vi "TestCloneAPI.vi"() -> ()   [LabVIEW 2014, in "NetworkImpairmentModule.lvlib"]
uses:
  NetworkImpairmentModule.lvlib
  PublicAPI/Arguments/Requests/dblTimeArray.ctl
  PublicAPI/Arguments/Requests/dblNetImpParams.ctl
  PublicAPI/Arguments/Requests/dblLossThreshold.ctl
  PublicAPI/Arguments/Broadcasts/dblNetworkTime.ctl
  PublicAPI/Arguments/Broadcasts/dblPktLoss.ctl
  <userlib>/NIST/ModuleAdminLib/ModuleAdmin/ModuleAdmin.lvclass
  PublicAPI/Arguments/Broadcasts/clDidInit.ctl
  <userlib>/NIST/ModuleAdminLib/ModuleAdmin/ModuleAdmin.lvclass/ModuleAdmin.ctl
  PublicAPI/Arguments/Requests/clStopArgument.ctl
  PublicAPI/Arguments/Broadcasts/clStatUpdate.ctl
  PublicAPI/Arguments/Broadcasts/clErrorRpt.ctl
  <userlib>/NIST/ModuleAdminLib/ModuleAdmin/Accessors/Read CloneRegRef.vi
  <vilib>/Analysis/1siggen.llb/Ramp Pattern by Delta.vi
  <userlib>/NIST/ModuleAdminLib/CloneRegistration/CloneRegistration.lvclass
  <vilib>/Analysis/NI_AALBase.lvlib
panel:
  in  "Show Panel":bool=TRUE
  out "PluginPathReport":path
  in  "btnReadPathToNetImpairPlugin":bool
  in  "btnLoadNetImpairPlugin":bool
  in  "PluginPath":path=path "P:/Framework/NetworkImpairment/NetworkImpairmentPlugins/NetworkPlugin/NetworkPlugin.ini"
  in  "Delta":dbl=60.0
  in  "End":dbl=10.0
  in  "Start":dbl
  in  "btnGetPktLoss":bool
  in  "btnGetNetTime":bool
  out "dblPktLoss":T1
  out "dblNetTime":T2
  in  "btnReadLossThreshold":bool
  out "dblLossThresholdReport":T3
  in  "btnWriteLossThreshold":bool
  in  "dblLossThreshold":T3
  in  "btnReadNetImpParams":bool
  out "dblNetImpParamsReport":T4
  in  "btnWriteNetImpParams":bool
  in  "dblNetImpParams":T4=[[0.5], [0.1], [0.03], [0.95], [5.0]]
  in  "dblTimeArray":T5
  in  "btnWriteTime":bool
  in  "btnRemove":bool
  out "Status Log":string
  out "Active Modules (Array)":string[](array[string])
  in  "btnAdd":bool
  in  "btnStop":bool
  in  "Select Module":i32(ring)=-1 caption="Select Module to send Request" items=["All"=-1, "4140002"=4140002, "4140003"=4140003, "4140004"=4140004, "4140005"=4140005]
  # "Hidden"
  # "Visible"
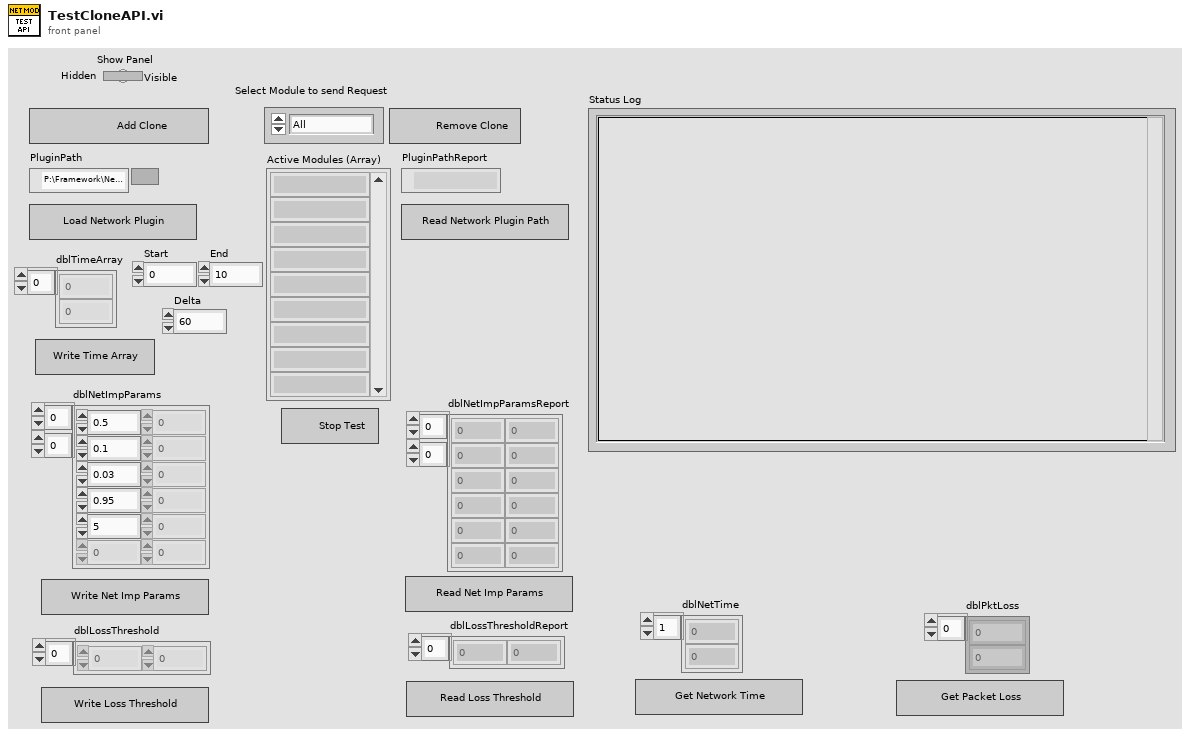
[diagram p1: front panel]
types:
  T1 = typedef "NetworkImpairmentModule.lvlib/dblPktLoss.ctl" = dbl[]
  T2 = typedef "NetworkImpairmentModule.lvlib/dblNetworkTime.ctl" = dbl[]
  T3 = typedef "NetworkImpairmentModule.lvlib/dblLossThreshold.ctl" = dbl[]
  T4 = typedef "NetworkImpairmentModule.lvlib/dblNetImpParams.ctl" = dbl[][]
  T5 = typedef "NetworkImpairmentModule.lvlib/dblTimeArray.ctl" = dbl[]
  T6 = typedef "NetworkImpairmentModule.lvlib/clBroadcastEvents.ctl" = cluster{"DidInit":refnum<user-event>, "StatusUpdate":refnum<user-event>, "ErrorReport":refnum<user-event>, "DidStop":refnum<user-event>, "ReadNetImpParams":refnum<user-event>, "ReadLossThreshold":refnum<user-event>, "GetNetworkTime":refnum<user-event>, "GetPktLoss":refnum<user-event>, "ReadPathToPlugin":refnum<user-event>}
  T7 = typedef "NetworkImpairmentModule.lvlib/clDidInit.ctl" = cluster{"Init?":bool, "ModuleAdmin":refnum<class "ModuleAdmin.lvclass">}
  T8 = typedef "NetworkImpairmentModule.lvlib/clStopArgument.ctl" = cluster{"Exit via Stop Module Req?":bool, "Wait for Module to stop?":bool, "ModuleAdmin":refnum<class "ModuleAdmin.lvclass">}
  T9 = typedef "NetworkImpairmentModule.lvlib/clStatUpdate.ctl" = cluster{"Status":string}
  T10 = typedef "NetworkImpairmentModule.lvlib/clErrorRpt.ctl" = cluster{"error":errorcluster, "AdditionalInfo":string}
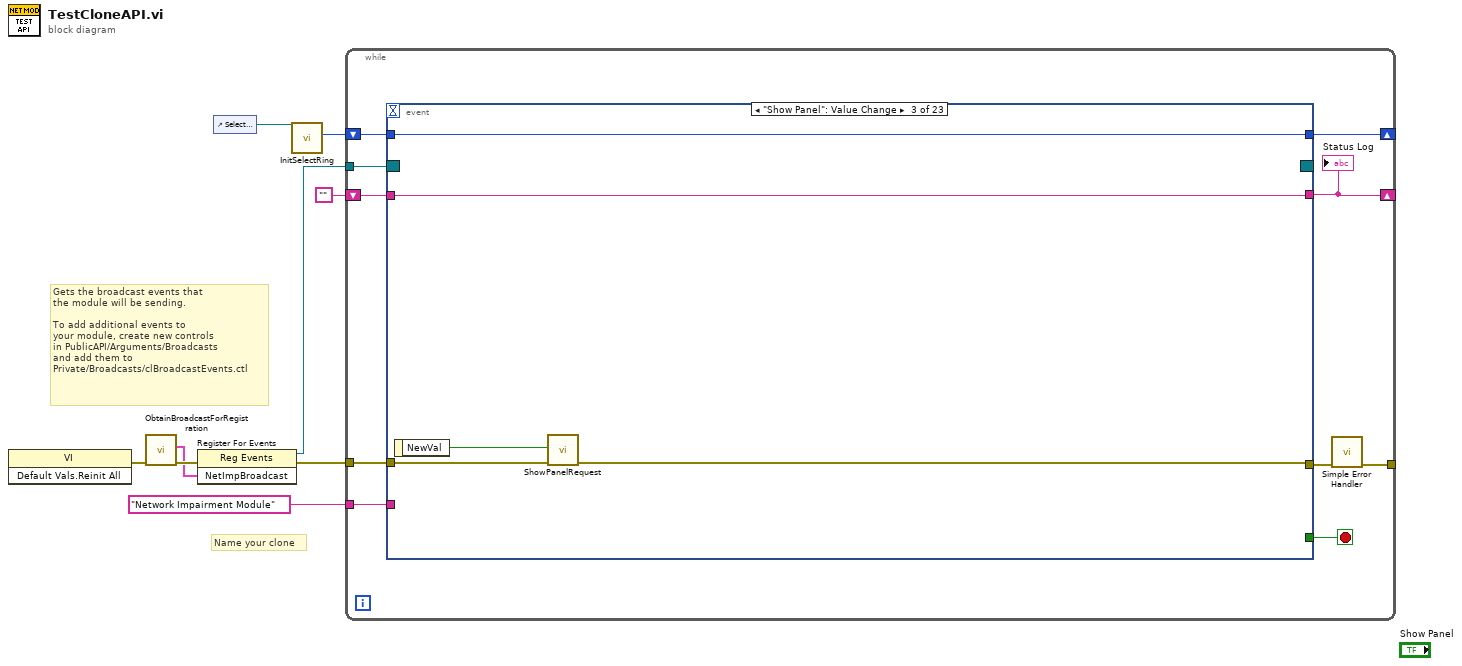
[diagram p0: block diagram]
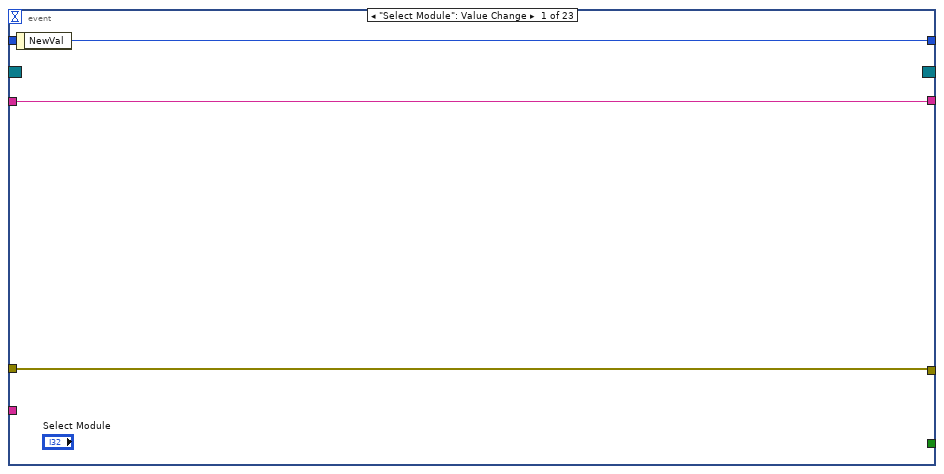
[diagram p2: hidden frame]
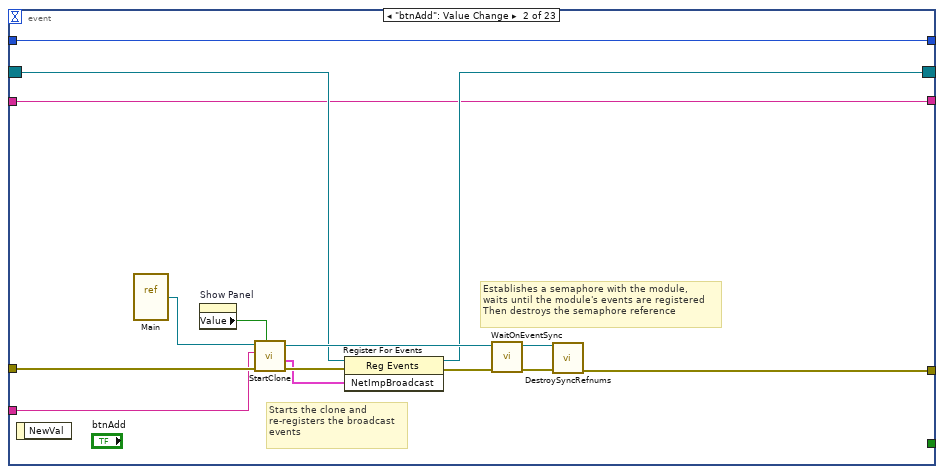
[diagram p3: hidden frame]
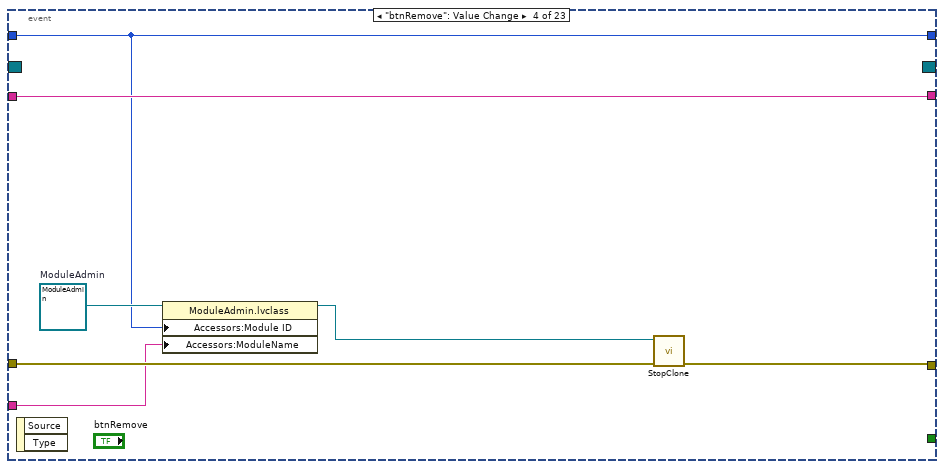
[diagram p4: hidden frame]
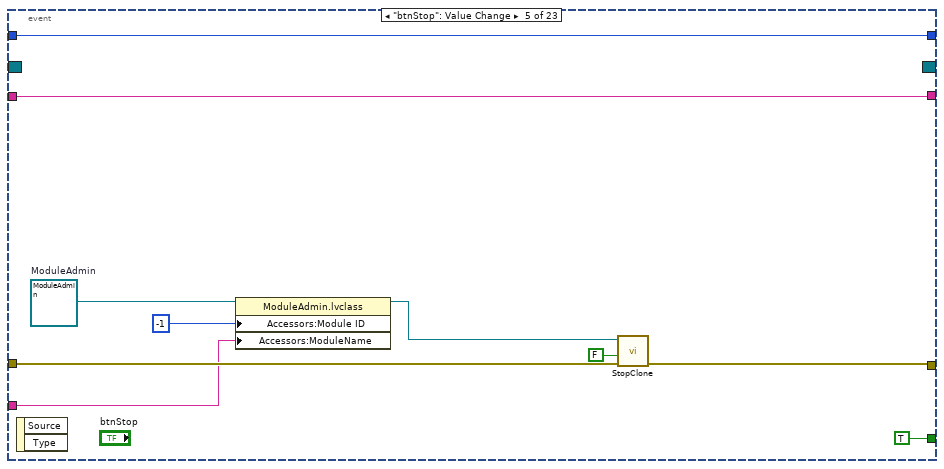
[diagram p5: hidden frame]
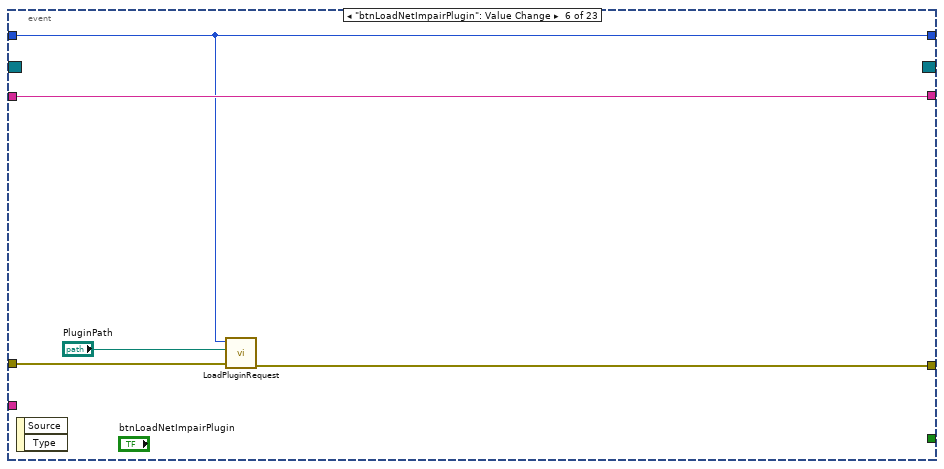
[diagram p6: hidden frame]
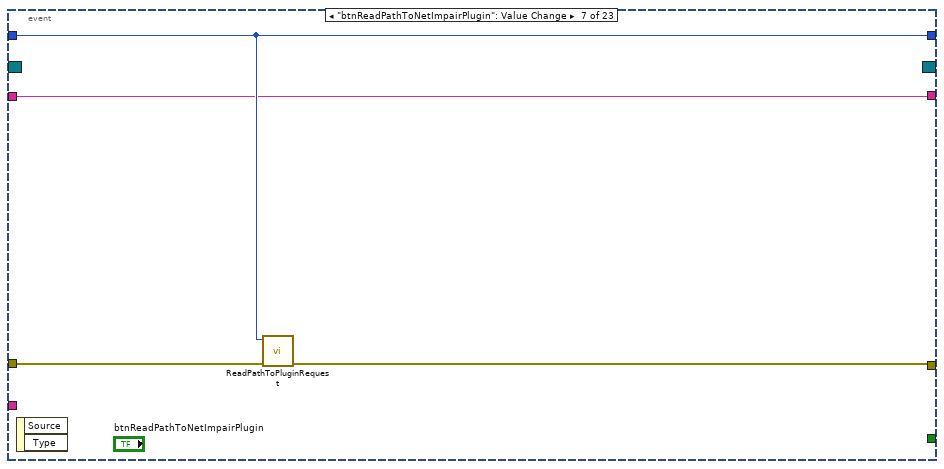
[diagram p7: hidden frame]
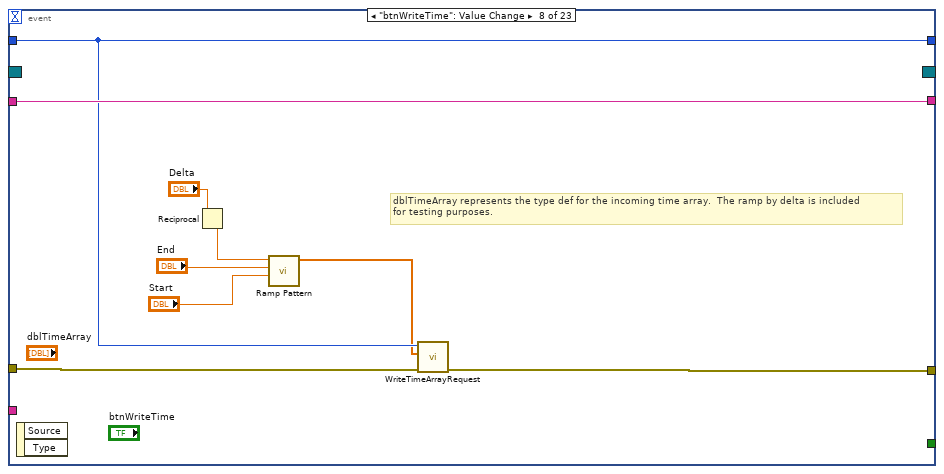
[diagram p8: hidden frame]
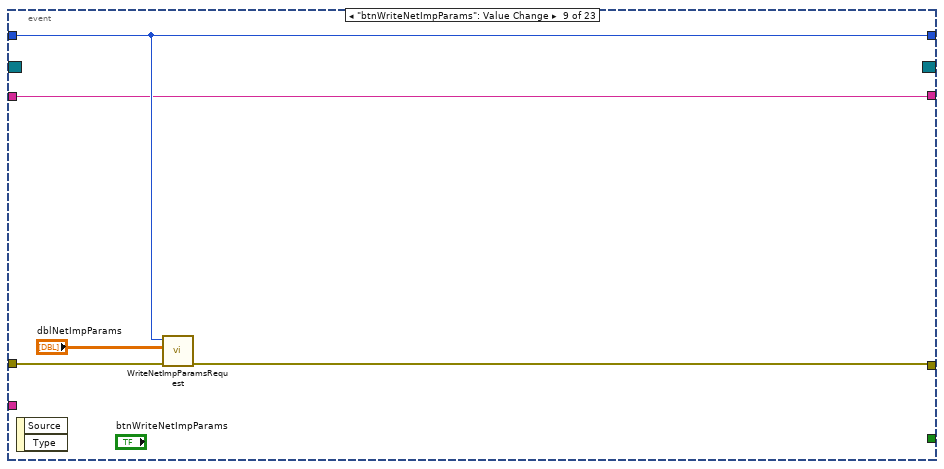
[diagram p9: hidden frame]
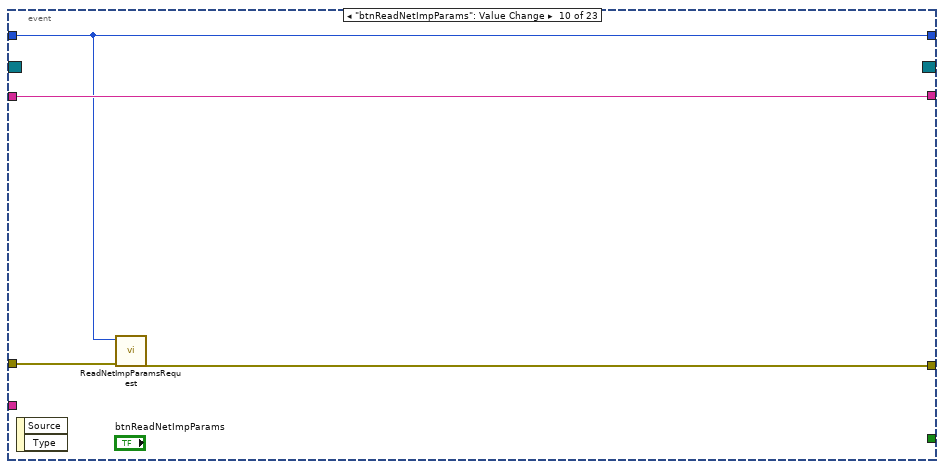
[diagram p10: hidden frame]
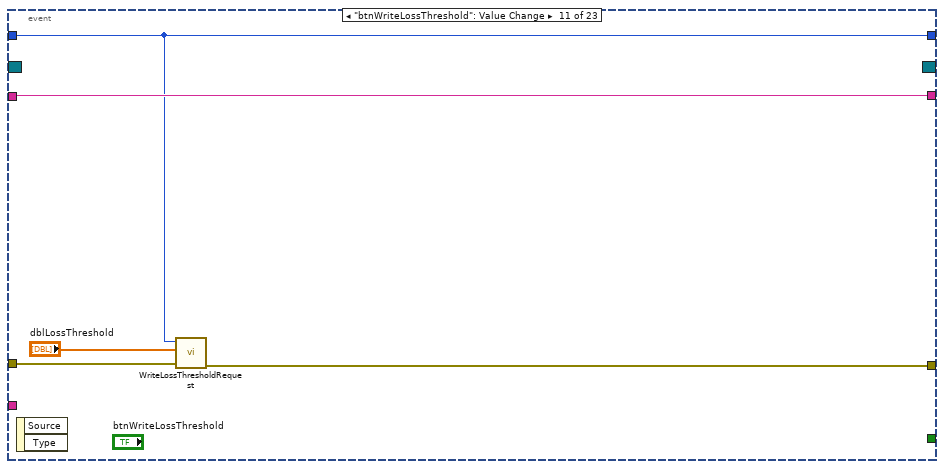
[diagram p11: hidden frame]
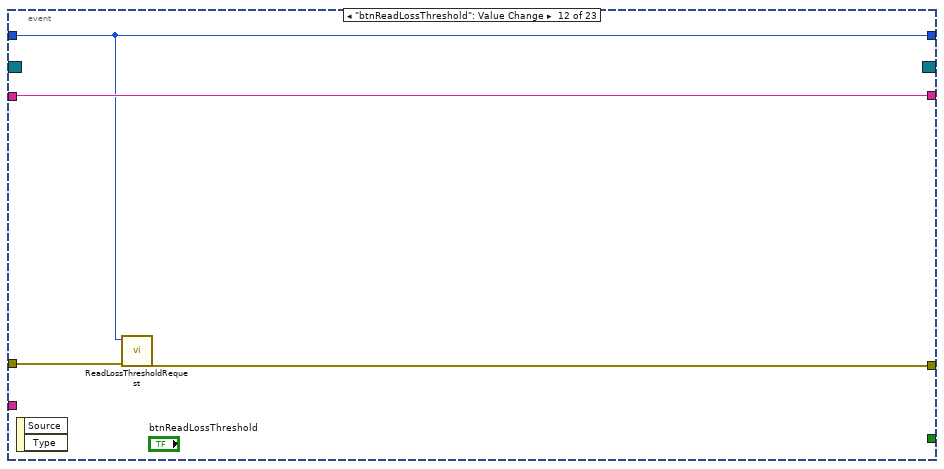
[diagram p12: hidden frame]
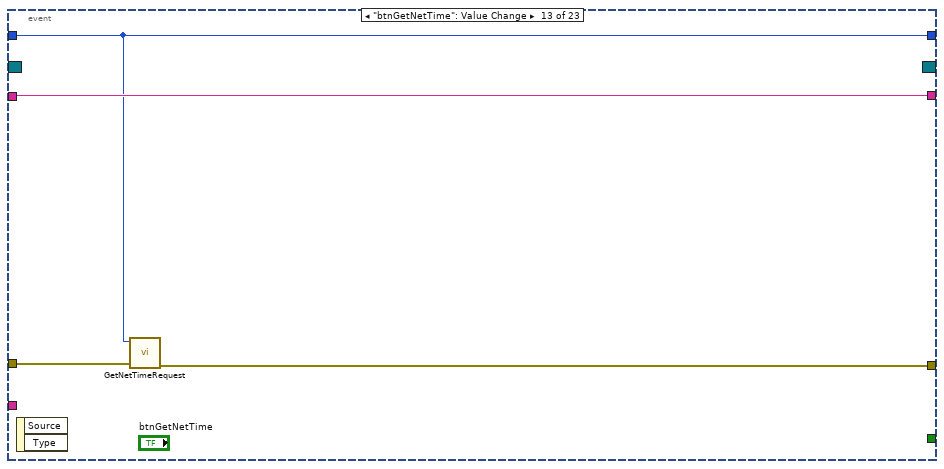
[diagram p13: hidden frame]
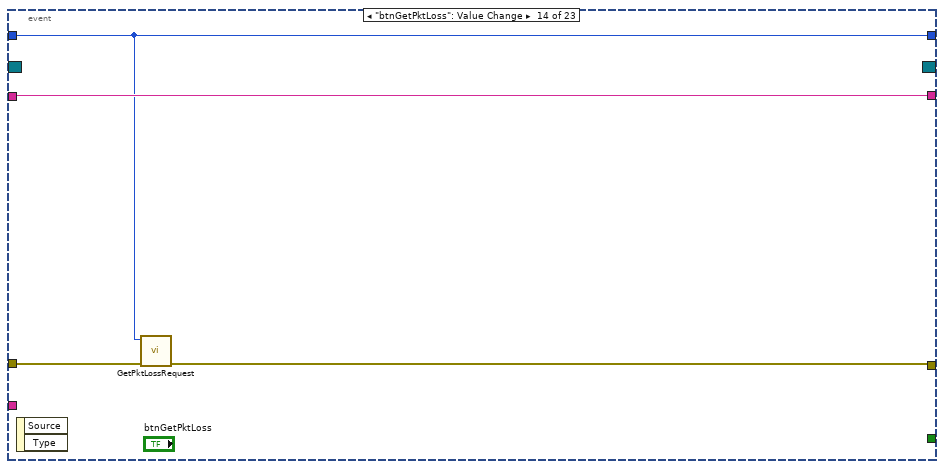
[diagram p14: hidden frame]
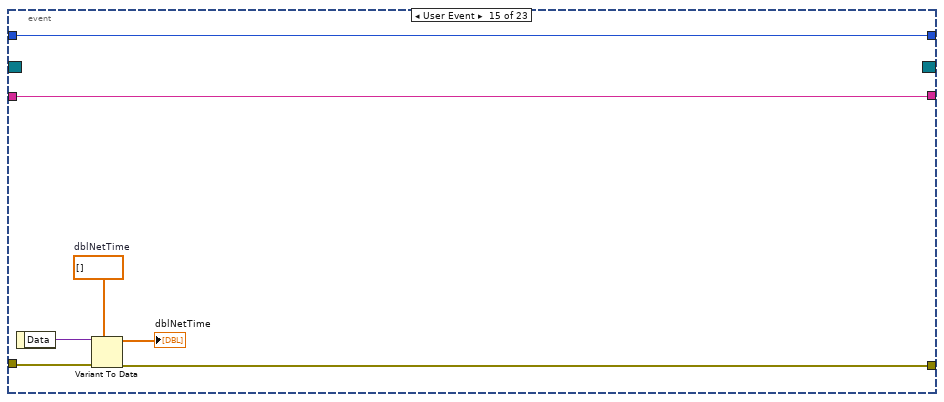
[diagram p15: hidden frame]
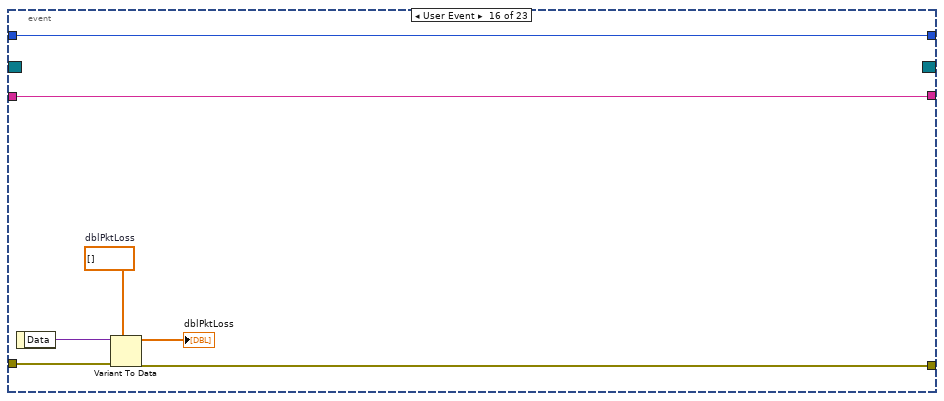
[diagram p16: hidden frame]
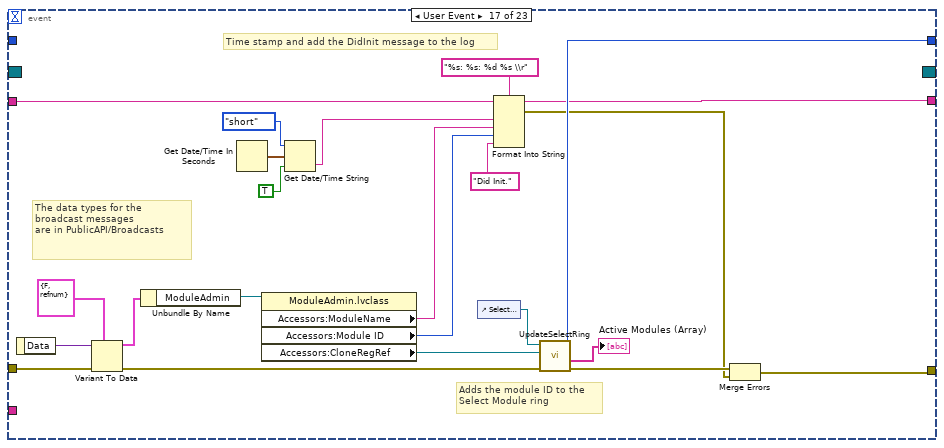
[diagram p17: hidden frame]
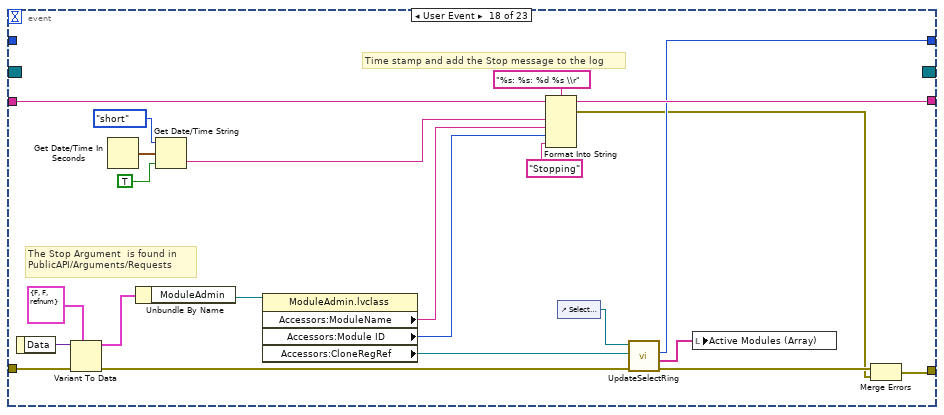
[diagram p18: hidden frame]
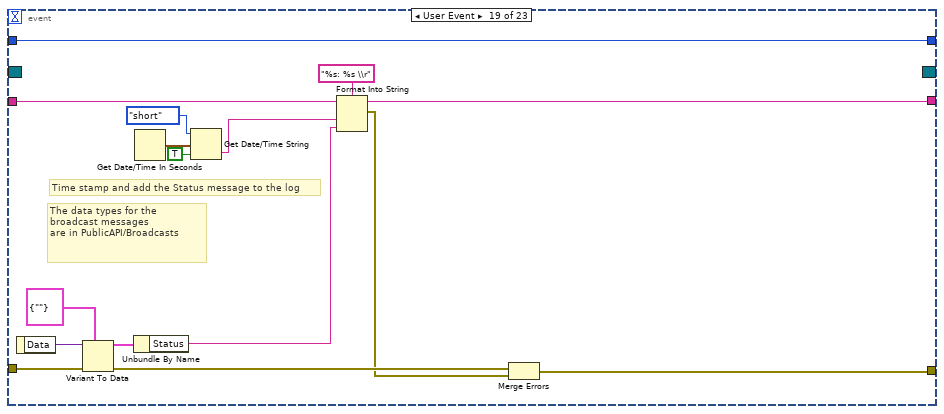
[diagram p19: hidden frame]
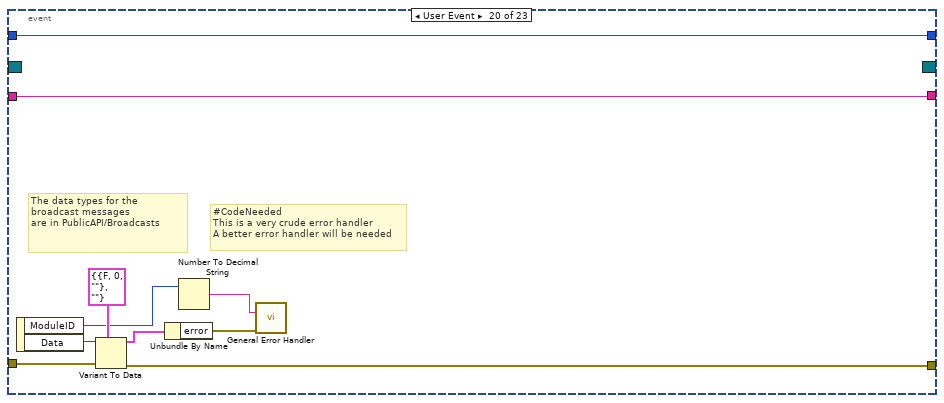
[diagram p20: hidden frame]
diagram:
  # "Name your clone"
  # "Gets the broadcast events that\nthe module will be sending.\n\nTo add additional events to\nyour module, create new controls\nin PublicAPI/Arguments/Broadcasts\nand add them to\nPrivate/Broadcasts/clBroadcastEvents.ctl"
  n1 = invoke class="VI" method="Default Vals.Reinit All"() -> (error out=w7:errorcluster)  [unwired: 3 in, 2 out]
  n2 = call "ObtainBroadcastForRegistration.vi"("error in (no error)"=w7) -> ("error out"=w6:errorcluster, "NetImpBroadcast"=w5:T6)  [unwired: 9 in]
  n3 = register-events(error in=w6, w5) -> (reference out=w3:refnum<event-registration>, error out=w4:errorcluster)  [unwired: 1 in]
  n4 = control-ref of="Select Module"() -> (w9:refnum<vi>)
  n5 = call "InitSelectRing.vi"("Ring Refnum"=w9) -> ("Module Ring Value"=w8:i32)  [unwired: 9 in, 1 out]
  n6 = while {
    shift-right: [w18] -> _
    shift-left: w8 -> [w19]
    tunnel: w4 -> [w16]
    tunnel: w3 -> [w13]
    tunnel: [w14] -> _
    shift-right: [w12] -> _
    shift-left: "" -> [w11]
    tunnel: "Network Impairment Module" ("ModuleName") -> [w10]
    stop <- w17 stop-if-true
    n7 = event shown="[2] \"Show Panel\": Value Change" {
      selector: w13 -> [_ w28 _ _ _ _ _ _ _ _ _ _ _ _ _ _ _ _ _ _ _ _ _]
      dyn-events: [_ w27 _ _ _ _ _ _ _ _ _ _ _ _ _ _ _ _ _ _ _ _ _] -> _
      timeout: _ -> [_ _ _ _ _ _ _ _ _ _ _ _ _ _ _ _ _ _ _ _ _ _ _]
      tunnel: w19 -> [_ w37 w41 w44 w59 w60 w66 w75 w80 w83 w87 w92 w96 w100 w104 w111 _ _ w179 w181 w192 w197 w205]
      tunnel: [w22 w37 w41 w44 w59 w60 w66 w75 w80 w83 w87 w92 w96 w100 w104 w111 w135 w150 w179 w181 w192 w197 w205] -> w18
      tunnel: [_ _ _ _ TRUE _ _ _ _ _ _ _ _ _ _ _ _ _ _ _ _ _ _] -> w17
      tunnel: w16 -> [w20 w36 w40 w48 w57 w63 w68 w76 w82 w86 w91 w95 w99 w103 w110 w117 w140 w159 w176 w188 w195 w202 w210]
      tunnel: [w20 w29 w38 w47 w55 w62 w67 w74 w78 w85 w90 w94 w98 w102 w107 w114 w124 w147 w167 w187 w194 w201 w208] -> w15
      tunnel: [w21 w25 w42 w49 w54 w64 w65 w77 w79 w84 w89 w93 w97 w101 w105 w112 w128 w156 w170 w180 w191 w198 w204] -> w12
      tunnel: w11 -> [w21 w25 w42 w49 w54 w64 w65 w77 w79 w84 w89 w93 w97 w101 w105 w112 w127 w157 w178 w180 w191 w198 w204]
      tunnel: w10 -> [_ w24 _ w45 w51 _ _ _ _ _ _ _ _ _ _ _ _ _ _ _ _ _ _]
      event "Select Module": Value Change {
        n8 = event-data() -> ("NewVal"=w22:i32)  [unwired: 1 in]
      }
      event "btnAdd": Value Change {
        # "Establishes a semaphore with the module,\nwaits until the module's events are registered\nThen destroys the semaphore reference"
        # "Starts the clone and\nre-registers the broadcast \nevents"
        n9 = event-data() -> ()  [unwired: 1 in, 1 out]
        n10 = vi-ref "Main.vi"() -> (w26:refnum<vi>)
        n11 = property on="Show Panel" class="Bool (strict)"() -> ("Value"=w23:bool)  [unwired: 2 in, 2 out]
        n12 = call "StartClone.vi"("ShowPanel? (f)"=w23, "error in (no error)"=w36, "ModuleName"=w24, "VI Refnum"=w26) -> ("error out"=w35:errorcluster, "clBroadcastEvents"=w30:T6, "ModuleAdmin"=w32:refnum<class "ModuleAdmin.lvclass">)  [unwired: 5 in]
        n13 = register-events(reference=w28, error in=w35, w30) -> (reference out=w27:refnum<event-registration>, error out=w34:errorcluster)
        n14 = call <userlib>:"WaitOnEventSync.vi"("error in (no error)"=w34, "ModuleAdmin"=w32) -> ("error out"=w33:errorcluster, "ModuleAdmin"=w31:refnum<class "ModuleAdmin.lvclass">)  [unwired: 8 in]
        n15 = call <userlib>:"DestroySyncRefnums.vi"("error in (no error)"=w33, "ModuleAdmin"=w31) -> ("error out"=w29:errorcluster)  [unwired: 9 in]
      }
      event "Show Panel": Value Change {
        n16 = event-data() -> ("NewVal"=w39:bool)  [unwired: 1 in]
        n17 = call "ShowPanelRequest.vi"("error in (no error)"=w40, "ShowPanel?"=w39) -> ("error out"=w38:errorcluster)  [unwired: 9 in]
      }
      event "btnRemove": Value Change {
        w46 = refnum<class "ModuleAdmin.lvclass"> refnum  # ModuleAdmin
        n18 = event-data() -> ()  [unwired: 1 in, 2 out]
        n19 = property class="ModuleAdmin.lvclass"(reference=w46, "Accessors:Module ID"=w44, "Accessors:ModuleName"=w45) -> (reference out=w43:refnum<class "ModuleAdmin.lvclass">)  [unwired: 1 in, 1 out]
        n20 = call "StopClone.vi"("error in (no error)"=w48, "ModuleAdmin"=w43) -> ("error out"=w47:errorcluster)  [unwired: 9 in]
      }
      event "btnStop": Value Change {
        w53 = refnum<class "ModuleAdmin.lvclass"> refnum  # ModuleAdmin
        n21 = event-data() -> ()  [unwired: 1 in, 2 out]
        n22 = property class="ModuleAdmin.lvclass"(reference=w53, "Accessors:Module ID"=-1 ("Module ID"), "Accessors:ModuleName"=w51) -> (reference out=w50:refnum<class "ModuleAdmin.lvclass">)  [unwired: 1 in, 1 out]
        n23 = call "StopClone.vi"("error in (no error)"=w57, "Wait for Module to stop?"=FALSE, "ModuleAdmin"=w50) -> ("error out"=w55:errorcluster)  [unwired: 8 in]
      }
      event "btnLoadNetImpairPlugin": Value Change {
        n24 = event-data() -> ()  [unwired: 1 in, 2 out]
        n25 = call "LoadPluginRequest.vi"("error in (no error)"=w63, "PathToPlugin"="PluginPath", "ModuleID"=w60) -> ("error out"=w62:errorcluster)  [unwired: 8 in]
      }
      event "btnReadPathToNetImpairPlugin": Value Change {
        n26 = event-data() -> ()  [unwired: 1 in, 2 out]
        n27 = call "ReadPathToPluginRequest.vi"("error in (no error)"=w68, "ModuleID"=w66) -> ("error out"=w67:errorcluster)  [unwired: 9 in]
      }
      event "btnWriteTime": Value Change {
        # "dblTimeArray represents the type def for the incoming time array.  The ramp by delta is included\nfor testing purposes."
        n28 = event-data() -> ()  [unwired: 1 in, 2 out]
        n29 = Reciprocal(x="Delta") -> (1/x=w69:dbl)
        n30 = call-poly <vilib>:"Ramp Pattern.vi"("start"="Start", "end"="End", "delta"=w69) -> ("Ramp Pattern"=w70:dbl[])  [unwired: 6 in, 2 out]
        n31 = call "WriteTimeArrayRequest.vi"("error in (no error)"=w76, "TimeArray"=w70, "Module ID"=w75) -> ("error out"=w74:errorcluster)  [unwired: 8 in]
      }
      event "btnWriteNetImpParams": Value Change {
        n32 = event-data() -> ()  [unwired: 1 in, 2 out]
        n33 = call "WriteNetImpParamsRequest.vi"("error in (no error)"=w82, "dblNetImpParams"="dblNetImpParams", "ModuleID"=w80) -> ("error out"=w78:errorcluster)  [unwired: 8 in]
      }
      event "btnReadNetImpParams": Value Change {
        n34 = event-data() -> ()  [unwired: 1 in, 2 out]
        n35 = call "ReadNetImpParamsRequest.vi"("error in (no error)"=w86, "ModuleID"=w83) -> ("error out"=w85:errorcluster)  [unwired: 9 in]
      }
      event "btnWriteLossThreshold": Value Change {
        n36 = event-data() -> ()  [unwired: 1 in, 2 out]
        n37 = call "WriteLossThresholdRequest.vi"("error in (no error)"=w91, "dblLossThreshold"="dblLossThreshold", "ModuleID"=w87) -> ("error out"=w90:errorcluster)  [unwired: 8 in]
      }
      event "btnReadLossThreshold": Value Change {
        n38 = event-data() -> ()  [unwired: 1 in, 2 out]
        n39 = call "ReadLossThresholdRequest.vi"("error in (no error)"=w95, "ModuleID"=w92) -> ("error out"=w94:errorcluster)  [unwired: 9 in]
      }
      event "btnGetNetTime": Value Change {
        n40 = event-data() -> ()  [unwired: 1 in, 2 out]
        n41 = call "GetNetTimeRequest.vi"("error in (no error)"=w99, "ModuleID"=w96) -> ("error out"=w98:errorcluster)  [unwired: 9 in]
      }
      event "btnGetPktLoss": Value Change {
        n42 = event-data() -> ()  [unwired: 1 in, 2 out]
        n43 = call "GetPktLossRequest.vi"("error in (no error)"=w103, "ModuleID"=w100) -> ("error out"=w102:errorcluster)  [unwired: 9 in]
      }
      event User Event {
        w106 = T2 []  # dblNetTime
        n44 = event-data() -> ("Data"=w109:variant)  [unwired: 1 in]
        n45 = Variant To Data(error in=w110, type=w106, Variant=w109) -> (data=→"dblNetTime":T2, error out=w107:errorcluster)
      }
      event User Event {
        w113 = T1 []  # dblPktLoss
        n46 = event-data() -> ("Data"=w116:variant)  [unwired: 1 in]
        n47 = Variant To Data(error in=w117, type=w113, Variant=w116) -> (data=→"dblPktLoss":T1, error out=w114:errorcluster)
      }
      event User Event {
        # "Adds the module ID to the \nSelect Module ring"
        # "Time stamp and add the DidInit message to the log"
        # "The data types for the broadcast messages\nare in PublicAPI/Broadcasts"
        n48 = event-data() -> ("Data"=w139:variant)  [unwired: 1 in]
        n49 = Variant To Data(error in=w140, type=T7 {"Init?"=FALSE, "ModuleAdmin"=refnum} ("clDidInit"), Variant=w139) -> (data=w132:T7, error out=w137:errorcluster)
        n50 = Unbundle By Name(w132) -> ("ModuleAdmin"=w121:refnum<class "ModuleAdmin.lvclass">)
        n51 = Get Date/Time In Seconds() -> (seconds since 1Jan1904=w130:timestamp)
        n52 = property class="ModuleAdmin.lvclass"(reference=w121) -> ("Accessors:ModuleName"=w120:string, "Accessors:Module ID"=w119:i32, "Accessors:CloneRegRef"=w118:refnum<data-value>)  [unwired: 1 in, 2 out]
        n53 = Get Date/Time String(date format (0)=enum16{"short", "long", "abbreviated"}."short", seconds (now)=w130, want seconds? (F)=TRUE) -> (time string=w133:string)  [unwired: 1 out]
        n54 = control-ref of="Select Module"() -> (w136:refnum<vi>)
        n55 = Format Into String(format string="%s: %s: %d %s \\r", initial string=w127, w133, w120, w119, "Did Init.") -> (resulting string=w128:string, error out=w125:errorcluster)  [unwired: 1 in]
        n56 = call "UpdateSelectRing.vi"("error in (no error)"=w137, "CloneRegRef"=w118, "Ring Refnum"=w136) -> ("error out"=w126:errorcluster, "ActiveModules"=→"Active Modules (Array)":string[], "Module Ring Value"=w135:i32)  [unwired: 6 in]
        n57 = Merge Errors(w126, w125) -> (w124:errorcluster)
      }
      event User Event {
        # "Time stamp and add the Stop message to the log"
        # "The Stop Argument  is found in\nPublicAPI/Arguments/Requests"
        n58 = event-data() -> ("Data"=w158:variant)  [unwired: 1 in]
        n59 = Variant To Data(error in=w159, type=T8 {"Exit via Stop Module Req?"=FALSE, "Wait for Module to stop?"=FALSE, "ModuleAdmin"=refnum} ("Stop Argument"), Variant=w158) -> (data=w154:T8, error out=w153:errorcluster)
        n60 = Get Date/Time In Seconds() -> (seconds since 1Jan1904=w161:timestamp)
        n61 = Unbundle By Name(w154) -> ("ModuleAdmin"=w143:refnum<class "ModuleAdmin.lvclass">)
        n62 = Get Date/Time String(date format (0)=enum16{"short", "long", "abbreviated"}."short", seconds (now)=w161, want seconds? (F)=TRUE) -> (time string=w163:string)  [unwired: 1 out]
        n63 = property class="ModuleAdmin.lvclass"(reference=w143) -> ("Accessors:ModuleName"=w142:string, "Accessors:Module ID"=w141:i32, "Accessors:CloneRegRef"=w144:refnum<data-value>)  [unwired: 1 in, 2 out]
        n64 = Format Into String(format string="%s: %s: %d %s \\r", initial string=w157, w163, w142, w141, "Stopping") -> (resulting string=w156:string, error out=w148:errorcluster)  [unwired: 1 in]
        n65 = control-ref of="Select Module"() -> (w152:refnum<vi>)
        n66 = call "UpdateSelectRing.vi"("error in (no error)"=w153, "CloneRegRef"=w144, "Ring Refnum"=w152) -> ("error out"=w149:errorcluster, "ActiveModules"=w151:string[], "Module Ring Value"=w150:i32)  [unwired: 6 in]
        n67 = local write "Active Modules (Array)"(w151) -> ()
        n68 = Merge Errors(w149, w148) -> (w147:errorcluster)
      }
      event User Event {
        # "Time stamp and add the Status message to the log"
        # "The data types for the broadcast messages\nare in PublicAPI/Broadcasts"
        n69 = event-data() -> ("Data"=w175:variant)  [unwired: 1 in]
        n70 = Variant To Data(error in=w176, type=T9 {"Status"=""} ("clStatUpdate"), Variant=w175) -> (data=w173:T9, error out=w169:errorcluster)
        n71 = Unbundle By Name(w173) -> ("Status"=w171:string)
        n72 = Get Date/Time In Seconds() -> (seconds since 1Jan1904=w172:timestamp)
        n73 = Get Date/Time String(date format (0)=enum16{"short", "long", "abbreviated"}."short", seconds (now)=w172, want seconds? (F)=TRUE) -> (time string=w164:string)  [unwired: 1 out]
        n74 = Format Into String(format string="%s: %s \\r", initial string=w178, w164, w171) -> (resulting string=w170:string, error out=w168:errorcluster)  [unwired: 1 in]
        n75 = Merge Errors(w169, w168) -> (w167:errorcluster)
      }
      event User Event {
        # "#CodeNeeded\nThis is a very crude error handler\nA better error handler will be needed"
        # "The data types for the broadcast messages\nare in PublicAPI/Broadcasts"
        n76 = event-data() -> ("ModuleID"=w184:i32, "Data"=w189:variant)  [unwired: 1 in]
        n77 = Variant To Data(error in=w188, type=T10 {"error"={"status"=FALSE, "code"=0, "source"=""}, "AdditionalInfo"=""} ("Cluster"), Variant=w189) -> (data=w185:T10, error out=w187:errorcluster)
        n78 = Unbundle By Name(w185) -> ("error"=w183:errorcluster)
        n79 = Number To Decimal String(number=w184) -> (decimal integer string=w182:string)  [unwired: 1 in]
        n80 = call <vilib>:"General Error Handler.vi"("[error source] (\" \")"=w182, "error in (no error)"=w183) -> ()  [unwired: 9 in, 5 out]
      }
      event User Event {
        n81 = event-data() -> ("Data"=w196:variant)  [unwired: 1 in]
        n82 = Variant To Data(error in=w195, type=path "", Variant=w196) -> (data=→"PluginPathReport":path, error out=w194:errorcluster)
      }
      event User Event {
        w200 = T4 []  # dblNetImpParams
        n83 = event-data() -> ("Data"=w203:variant)  [unwired: 1 in]
        n84 = Variant To Data(error in=w202, type=w200, Variant=w203) -> (data=→"dblNetImpParamsReport":T4, error out=w201:errorcluster)
      }
      event User Event {
        w206 = T3 []  # dblLossThreshold
        n85 = event-data() -> ("Data"=w209:variant)  [unwired: 1 in]
        n86 = Variant To Data(error in=w210, type=w206, Variant=w209) -> (data=→"dblLossThresholdReport":T3, error out=w208:errorcluster)
      }
    }
    "Status Log" <- w12
    n87 = call <vilib>:"Simple Error Handler.vi"("error in (no error)"=w15) -> ("error out"=w14:errorcluster)  [unwired: 4 in, 4 out]
  }
